vi "LeCroyAVG_Wait.vi"(7 "EXT AVG":bool, 8 "error in":errorcluster, 10 "Avg Num":i32=1, 11 "LeCroy":refnum<visa-resource-name>) -> (0 "error out":errorcluster, 3 "LeCroy":refnum<visa-resource-name>)   [LabVIEW 2022 SP3]
uses:
  <vilib>/Platform/TimedLoop/XDataNode/timing_clust.ctl
  <vilib>/Platform/TimedLoop/XDataNode/nitl_modes.ctl
  <vilib>/Platform/TimedLoop/XDataNode/wakeup.ctl
  <vilib>/Platform/TimedLoop/XDataNode/XDataNode.xnode
  <instrlib>/LeCroy Wave Series/LeCroy Wave Series.lvlib
  <vilib>/Platform/TimedLoop/XDataNode/XDNodeRunTimeDep.lvlib
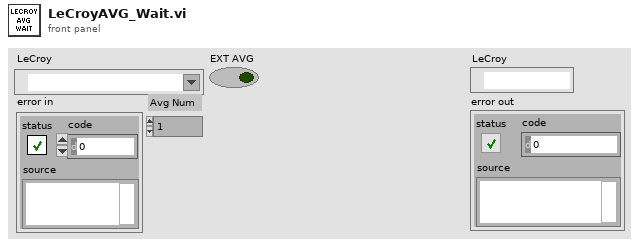
[diagram p1: front panel]
types:
  T1 = typedef "XDNodeRunTimeDep.lvlib/timing_clust.ctl" = cluster{"Expected End [f-1]":u64, "Actual End [f-1]":u64, "Finished Late? [f-1]":bool, "Expected End [i-1]":u64, "Actual End [i-1]":u64, "Finished Late? [i-1]":bool, "Expected Start [i]":u64, "Actual Start [i]":u64, "Expected Start [f]":u64, "Actual Start [f]":u64, "Source Name":string, "Structure Name":string, "Period":i64, "Deadline":i64, "Offset":i64, "Start":i64, "Priority":i32, "Timeout":i32, "Mode":T2, "Wakeup Reason":T3, "Error":errorcluster, "Source Type":string, "Secondary Source Type":string, "Global End Time":u64, "Global Start Time":u64, "Frame Duration":u64, "Iteration Duration":u64, "Assigned CPU":i32, "I/O Scan Engine Mode":u32}
  T2 = typedef "XDNodeRunTimeDep.lvlib/nitl_modes.ctl" = enum32{"No Change", "Process missed periods, maintain original phase", "Discard missed periods, maintain original phase", "Process missed periods, ignore original phase", "Discard missed periods, ignore original phase"}
  T3 = typedef "XDNodeRunTimeDep.lvlib/wakeup.ctl" = enum32{"Normal", "Aborted", "Asynchronous wakeup", "Timing source error", "Timed loop error", "Timeout"}
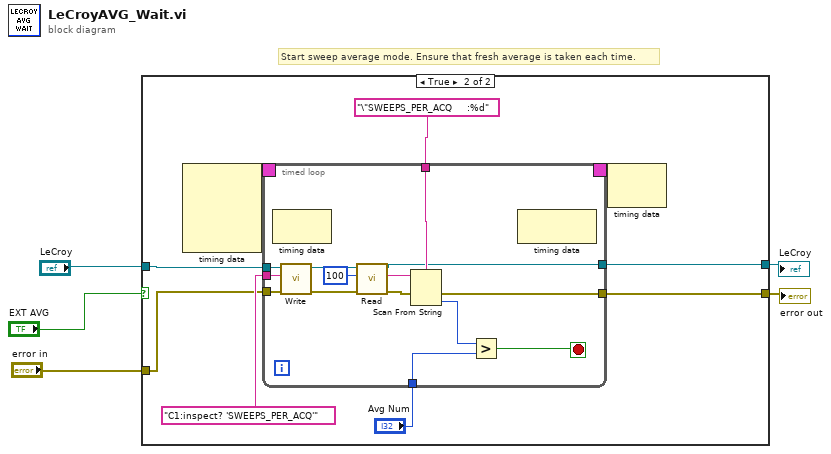
[diagram p0: block diagram]
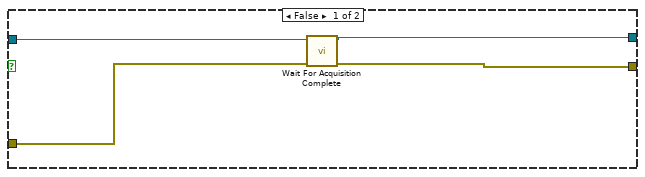
[diagram p2: hidden frame]
diagram:
  # "Start sweep average mode. Ensure that fresh average is taken each time."
  n1 = case shown="True" "EXT AVG" {
    tunnel: "LeCroy" -> [w9 w18]
    tunnel: "error in" -> [w7 w16]
    tunnel: [w8 w12] -> w3
    tunnel: [w6 w11] -> w2
    frame False {
      n2 = call <instrlib>:"Wait For Acquisition Complete.vi"("error in (no error)"=w7, "VISA resource name"=w9) -> ("error out"=w6:errorcluster, "VISA resource name out"=w8:refnum<visa-resource-name>)  [unwired: 7 in, 1 out]
    }
    frame True {
      n3 = node-c288() -> (w14:T1)  [unwired: 4 in]
      n4 = timed-loop {
        timing: w14 -> [_]
        timing-out: [_] -> w13
        tunnel: w18 -> [w27]
        tunnel: "C1:inspect? 'SWEEPS_PER_ACQ'" ("Write Buffer") -> [w26]
        tunnel: w16 -> [w25]
        tunnel: "\"SWEEPS_PER_ACQ     :%d" ("format string") -> [w24]
        tunnel: [w22] -> w12
        tunnel: [w21] -> w11
        tunnel: "Avg Num" -> [w19]
        stop <- w23 stop-if-true
        n5 = node-c288() -> ()  [unwired: 1 in, 1 out]
        n6 = call <instrlib>:"Write.vi"("error in (no error)"=w25, "Write Buffer"=w26, "VISA resource name"=w27) -> ("error out"=w31:errorcluster, "VISA resource name out"=w32:refnum<visa-resource-name>)  [unwired: 6 in, 1 out]
        n7 = call <instrlib>:"Read.vi"("error in (no error)"=w31, "Byte Count"=u32 100, "VISA resource name"=w32) -> ("error out"=w28:errorcluster, "Read Buffer"=w29:string, "VISA resource name out"=w22:refnum<visa-resource-name>)  [unwired: 5 in, 1 out]
        n8 = Scan From String(format string=w24, input string=w29, error in=w28) -> (error out=w21:errorcluster, output 1=w20:i32)  [unwired: 2 in, 2 out]
        n9 = Greater?(x=w20, y=w19) -> (0:w23:bool)
        n10 = node-c288() -> ()  [unwired: 1 in, 1 out]
      }
      n11 = node-c288(w13) -> ()  [unwired: 1 out]
    }
  }
  "LeCroy" <- w3
  "error out" <- w2
